vi "DJ Interface.vi"(10 "Owning VI":refnum<vi>, 11 "Shutdown Event":refnum<user-event>) -> ()   [LabVIEW 2020, in "User Interface.lvlib"]
doc: "Main control interface to Dataflow DJ. Also handles all keyboard shortcuts.\n\n<b>Execution System:</b> User Interface"
uses:
  User Interface.lvlib
  Custom Graphics/LED.Red.16px.ctl
  Custom Graphics/Slide.PlaybackPosition.ctl
  Custom Graphics/WaveformGraph.WaveformDisplay.ctl
  Custom Graphics/Knob.276px_Hole.ctl
  Custom Graphics/Button.Large.ctl
  Custom Graphics/PictRing.DeckLabel.ctl
  Custom Graphics/Button.Small.ctl
  <vilib>/Utility/miscctls.llb/LVCursorListTypeDef.ctl
  Packed Libraries/Audio Processing.lvlibp/Value Properties.ctl
  Packed Libraries/Messaging.lvlibp/Message Cluster.ctl
  Controls/Keyboard Shortcut.ctl
  Knob Fill.vi
  <vilib>/Utility/Data Type/Get Type Information.vi
  Packed Libraries/Messaging.lvlibp
  user32.dll
  Packed Libraries/Audio Processing.lvlibp
panel:
  in  "Deck1.Pitch":cluster{dbl, dbl}(slide) scale=30.0..-30.0
  in  "Channel2.EQMidKill":T1
  in  "Channel2.EQLowKill":T1
  in  "Channel2.EQHighKill":T1
  in  "Channel1.EQHighKill":T1
  in  "Channel1.EQMidKill":T1
  in  "Channel1.EQLowKill":T1
  in  "EffectUnit2.Effect3.Value2":dbl(knob) caption="DELAY" scale=0.0..1.0
  in  "EffectUnit2.Effect3.Value1":dbl(knob) caption="AMOUNT" scale=0.0..1.0
  in  "EffectUnit2.Effect2.Value2":dbl(knob)=16.0 caption="BIT DEPTH" step=1.0 scale=0.0..16.0
  in  "EffectUnit2.Effect2.Value1":dbl(knob)=1.0 caption="DECIMATION" step=1.0 scale=1.0..20.0
  in  "EffectUnit2.Effect1.Value2":dbl(knob) caption="SPEED" scale=0.0..0.1
  in  "EffectUnit2.Effect1.Value1":dbl(knob) caption="AMOUNT" scale=0.0..1.0
  in  "EffectUnit1.Effect3.Value2":dbl(knob) caption="DELAY" scale=0.0..1.0
  in  "EffectUnit1.Effect3.Value1":dbl(knob) caption="AMOUNT" scale=0.0..1.0
  in  "EffectUnit1.Effect2.Value2":dbl(knob)=16.0 caption="BIT DEPTH" step=1.0 scale=0.0..16.0
  in  "EffectUnit1.Effect2.Value1":dbl(knob)=1.0 caption="DECIMATION" step=1.0 scale=1.0..20.0
  in  "EffectUnit1.Effect1.Value2":dbl(knob) caption="SPEED" scale=0.0..0.1
  in  "EffectUnit1.Effect1.Value1":dbl(knob) caption="AMOUNT" scale=0.0..1.0
  in  "Channel2.EQLow":dbl(knob)=1.0 caption="LOW" scale=0.0..2.0
  in  "Channel2.EQMid":dbl(knob)=1.0 caption="MID" scale=0.0..2.0
  in  "Channel2.EQHigh":dbl(knob)=1.0 caption="HIGH" scale=0.0..2.0
  in  "Channel2.EQFilter":dbl(knob) caption="FILTER" scale=-1.025..1.025
  in  "Channel1.EQLow":dbl(knob)=1.0 caption="LOW" scale=0.0..2.0
  in  "Channel1.EQMid":dbl(knob)=1.0 caption="MID" scale=0.0..2.0
  in  "Channel1.EQHigh":dbl(knob)=1.0 caption="HIGH" scale=0.0..2.0
  in  "Channel1.EQFilter":dbl(knob) caption="FILTER" scale=-1.025..1.025
  in  "Channel2.Gain":dbl(knob)=1.0 caption="GAIN" scale=0.0..2.0
  in  "Mixer.Headphones":dbl(knob)=1.0 caption="PHONES" scale=0.0..1.0
  in  "Mixer.Master":dbl(knob)=1.0 caption="MASTER" scale=0.0..1.0
  in  "Channel1.Gain":dbl(knob)=1.0 caption="GAIN" scale=0.0..2.0
  out "Default Value Map":variant=variant("Channel1.EQFilter"=variant(dbl 0.0), "Channel1.EQHigh"=variant(dbl 1.0), "Channel1.EQLow"=variant(dbl 1.0), "Channel1.EQMid"=variant(dbl 1.0), "Channel1.Gain"=variant(dbl 1.0), "Channel1.Level"=variant(dbl 1.0), "Channel2.EQFilter"=variant(dbl 0.0), "Channel2.EQHigh"=variant(dbl 1.0), "Channel2.EQLow"=variant(dbl 1.0), "Channel2.EQMid"=variant(dbl 1.0), "Channel2.Gain"=variant(dbl 1.0), "Channel2.Level"=variant(dbl 1.0), "Deck1.Pitch"=variant(dbl 0.0), "Deck2.Pitch"=variant(dbl 0.0), "EffectUnit1.Effect1.Value1"=variant(dbl 0.0), "EffectUnit1.Effect1.Value2"=variant(dbl 0.0), "EffectUnit1.Effect2.Value1"=variant(dbl 1.0), "EffectUnit1.Effect2.Value2"=variant(dbl 16.0), "EffectUnit1.Effect3.Value1"=variant(dbl 0.0), "EffectUnit1.Effect3.Value2"=variant(dbl 0.0), "EffectUnit2.Effect1.Value1"=variant(dbl 0.0), "EffectUnit2.Effect1.Value2"=variant(dbl 0.0), "EffectUnit2.Effect2.Value1"=variant(dbl 1.0), "EffectUnit2.Effect2.Value2"=variant(dbl 16.0), "EffectUnit2.Effect3.Value1"=variant(dbl 0.0), "EffectUnit2.Effect3.Value2"=variant(dbl 0.0), "Mixer.Crossfader"=variant(dbl 0.0), "Mixer.Headphones"=variant(dbl 1.0), "Mixer.Master"=variant(dbl 1.0))
  in  "EffectUnit2.Effect3.Enable":T1
  in  "EffectUnit2.Effect2.Enable":T1
  in  "EffectUnit2.Effect1.Enable":T1
  in  "EffectUnit1.Effect3.Enable":T1
  in  "EffectUnit1.Effect2.Enable":T1
  in  "EffectUnit1.Effect1.Enable":T1
  in  "EffectUnit2.Effect3":u16(ring)=1 items=["CRUSHER", "ECHO", "FLANGER"]
  in  "EffectUnit2.Effect2":u16(ring) items=["CRUSHER", "ECHO", "FLANGER"]
  in  "EffectUnit2.Effect1":u16(ring)=2 items=["CRUSHER", "ECHO", "FLANGER"]
  in  "EffectUnit1.Effect3":u16(ring)=1 items=["CRUSHER", "ECHO", "FLANGER"]
  in  "EffectUnit1.Effect2":u16(ring) items=["CRUSHER", "ECHO", "FLANGER"]
  in  "EffectUnit1.Effect1":u16(ring)=2 items=["CRUSHER", "ECHO", "FLANGER"]
  in  "Deck2.DragDropPath":path
  in  "Deck1.DragDropPath":path
  in  "Deck2.PitchBendUp":T2
  in  "Deck2.PitchBendDown":T2
  in  "Channel2.HeadphoneOutput":T2
  in  "Channel1.HeadphoneOutput":T2
  in  "Deck1.PitchBendUp":T2
  in  "Deck1.PitchBendDown":T2
  in  "Deck2.Reverse":T3
  in  "Deck2.Backspin":T3
  in  "Deck2.Brake":T3
  in  "Deck2.Cue3":T3
  in  "Deck2.Cue2":T3
  in  "Deck2.Cue1":T3
  in  "Deck2.Play":T3
  in  "Deck1.Cue3":T3
  in  "Deck1.Cue2":T3
  in  "Deck1.Reverse":T3
  in  "Deck1.Backspin":T3
  in  "Deck1.Cue1":T3
  out "Deck2.Time":string
  in  "Deck2.PlaybackPosition":T4 scale=0.0..12805632.0
  out "Deck2.Waveform":T5
  out "Deck2.BPM":string
  out "Deck1.BPM":string
  in  "Deck1.Brake":T3
  out "Mixer.Right.LevelIndicator":u8(slide) scale=0.0..20.0
  out "Mixer.Left.LevelIndicator":u8(slide) scale=0.0..20.0
  in  "Deck1.Play":T3
  in  "Deck1.Jogwheel":T6 scale=0.0..79380.0
  in  "Deck2.Pitch":cluster{dbl, dbl}(slide) scale=30.0..-30.0
  out "Deck2.Title":string
  out "Deck1.Time":string
  out "Deck1.Title":string
  in  "Deck2.Jogwheel":T6 scale=0.0..79380.0
  in  "Channel2.Level":dbl(slide)=1.0 scale=0.0..1.0
  in  "Mixer.Crossfader":cluster{dbl, dbl}(slide) scale=-1.0..1.0
  in  "Channel1.Level":dbl(slide)=1.0 scale=0.0..1.0
  in  "Deck1.PlaybackPosition":T4 scale=0.0..12178944.0
  out "Deck1.Waveform":T5
  out "Deck1.JogwheelLabel":T7
  out "Deck2.JogwheelLabel":T7
  # "DECK 1\nCUE"
  # "DECK 2\nCUE"
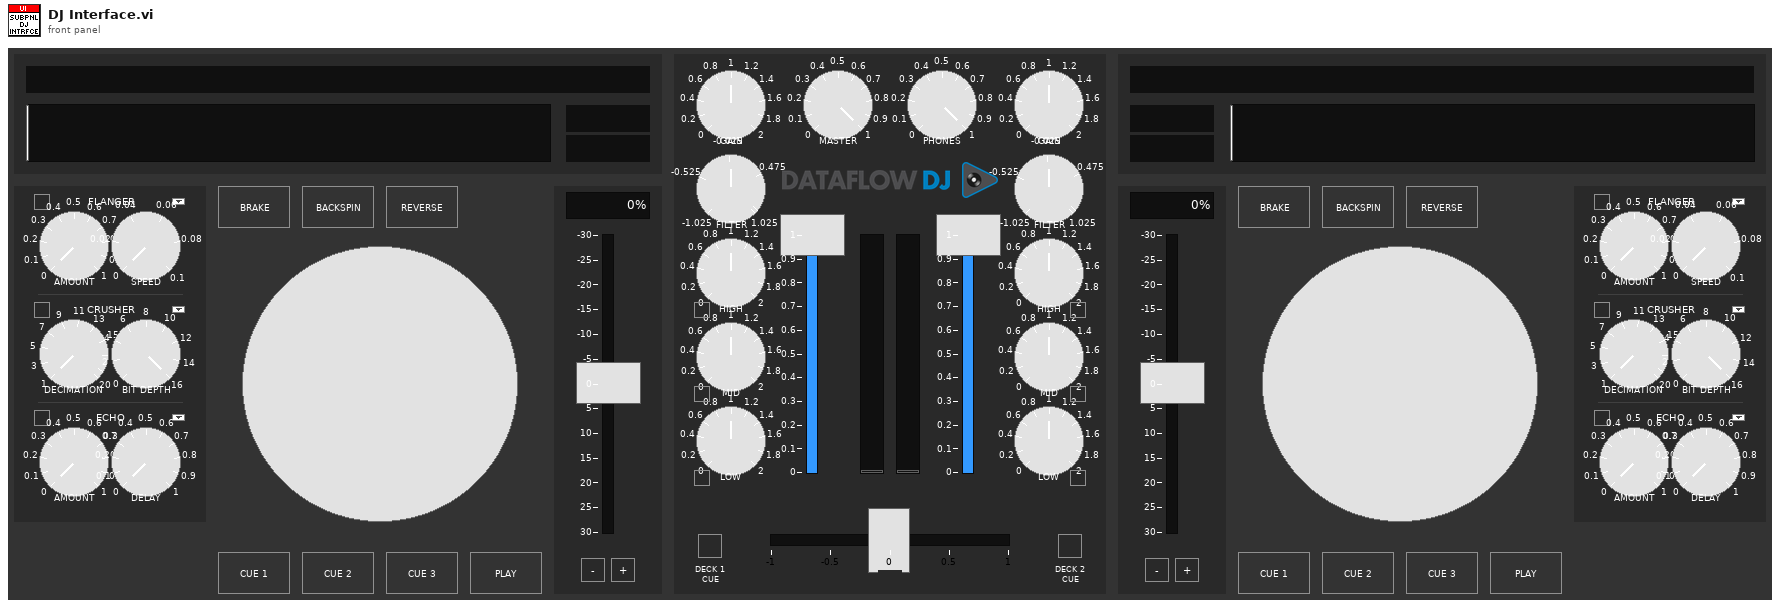
[diagram p1: front panel]
types:
  T1 = typedef "User Interface.lvlib/LED.Red.16px.ctl" = bool
  T2 = typedef "User Interface.lvlib/Button.Small.ctl" = bool
  T3 = typedef "User Interface.lvlib/Button.Large.ctl" = bool
  T4 = typedef "User Interface.lvlib/Slide.PlaybackPosition.ctl" = i32
  T5 = typedef "User Interface.lvlib/WaveformGraph.WaveformDisplay.ctl" = dbl[][]
  T6 = typedef "User Interface.lvlib/Knob.276px_Hole.ctl" = i32
  T7 = typedef "User Interface.lvlib/PictRing.DeckLabel.ctl" = u16
  T8 = typedef "LVCursorListTypeDef.ctl" = cluster{"Name":string, "Color":u32, "Style":u8, "Point Style":u8, "Name Visible":bool, "Allow Drag":bool, "Cursor Mode":u32, "Plot":i32, "Index":i32, "Position":cluster{"X":dbl, "Y":dbl}, "X Scale":u32, "Y Scale":u32, "Watch Plots":i32[], "Watch All Plots":bool, "Plot Area":i32, "Label Offset":cluster{"X":dbl, "Y":dbl}}[]
  T9 = typedef "Keyboard Shortcut.ctl" = cluster{"Keystroke":string, "Message Queue":string, "Event":string, "Target":string, "Data":variant}
  T10 = typedef "Audio Processing.lvlibp/Value Properties.ctl" = cluster{"Lower":dbl, "Upper":dbl, "Default":dbl, "Increment":dbl}
  T11 = typedef "Messaging.lvlib/Message Cluster.ctl" = cluster{"Event":string, "Source":string, "Target":string, "Data":variant}
  T12 = typedef "Messaging.lvlibp/Message Cluster.ctl" = cluster{"Event":string, "Source":string, "Target":string, "Data":variant}
  T13 = cluster{"type":i32, "KEYBDINPUT":cluster{"dx":i32, "dy":i32, "mouseData":i32, "dwFlags":i32, "time":i32, "dwExtraInfo":u32}}
  T14 = typedef "eventvkey.ctl" = enum16{"ASCII", "Enter", "Return", "Shift", "Ctrl", "Alt", "Cmd", "Opt", "Caps", "NumLock", "Clear", "Break", "Up", "Down", "Left", "Right", "Insert", "Delete", "Home", "End", "PageUp", "PageDown", "Escape", "Help", "Pause", "ScrollLock", "F1", "F2", "F3", "F4", "F5", "F6", "F7", "F8", "F9", "F10", "F11", "F12", "F13", "F14", "F15", "F16", "F17", "F18", "F19", "F20", "F21", "F22", "F23", "F24", "Play", "VolumeUp", "VolumeDown", "Mute", "Two Byte Char"}
  T15 = cluster{"Shift":bool, "Ctrl":bool, "Alt":bool, "Cmd":bool, "Opt":bool}
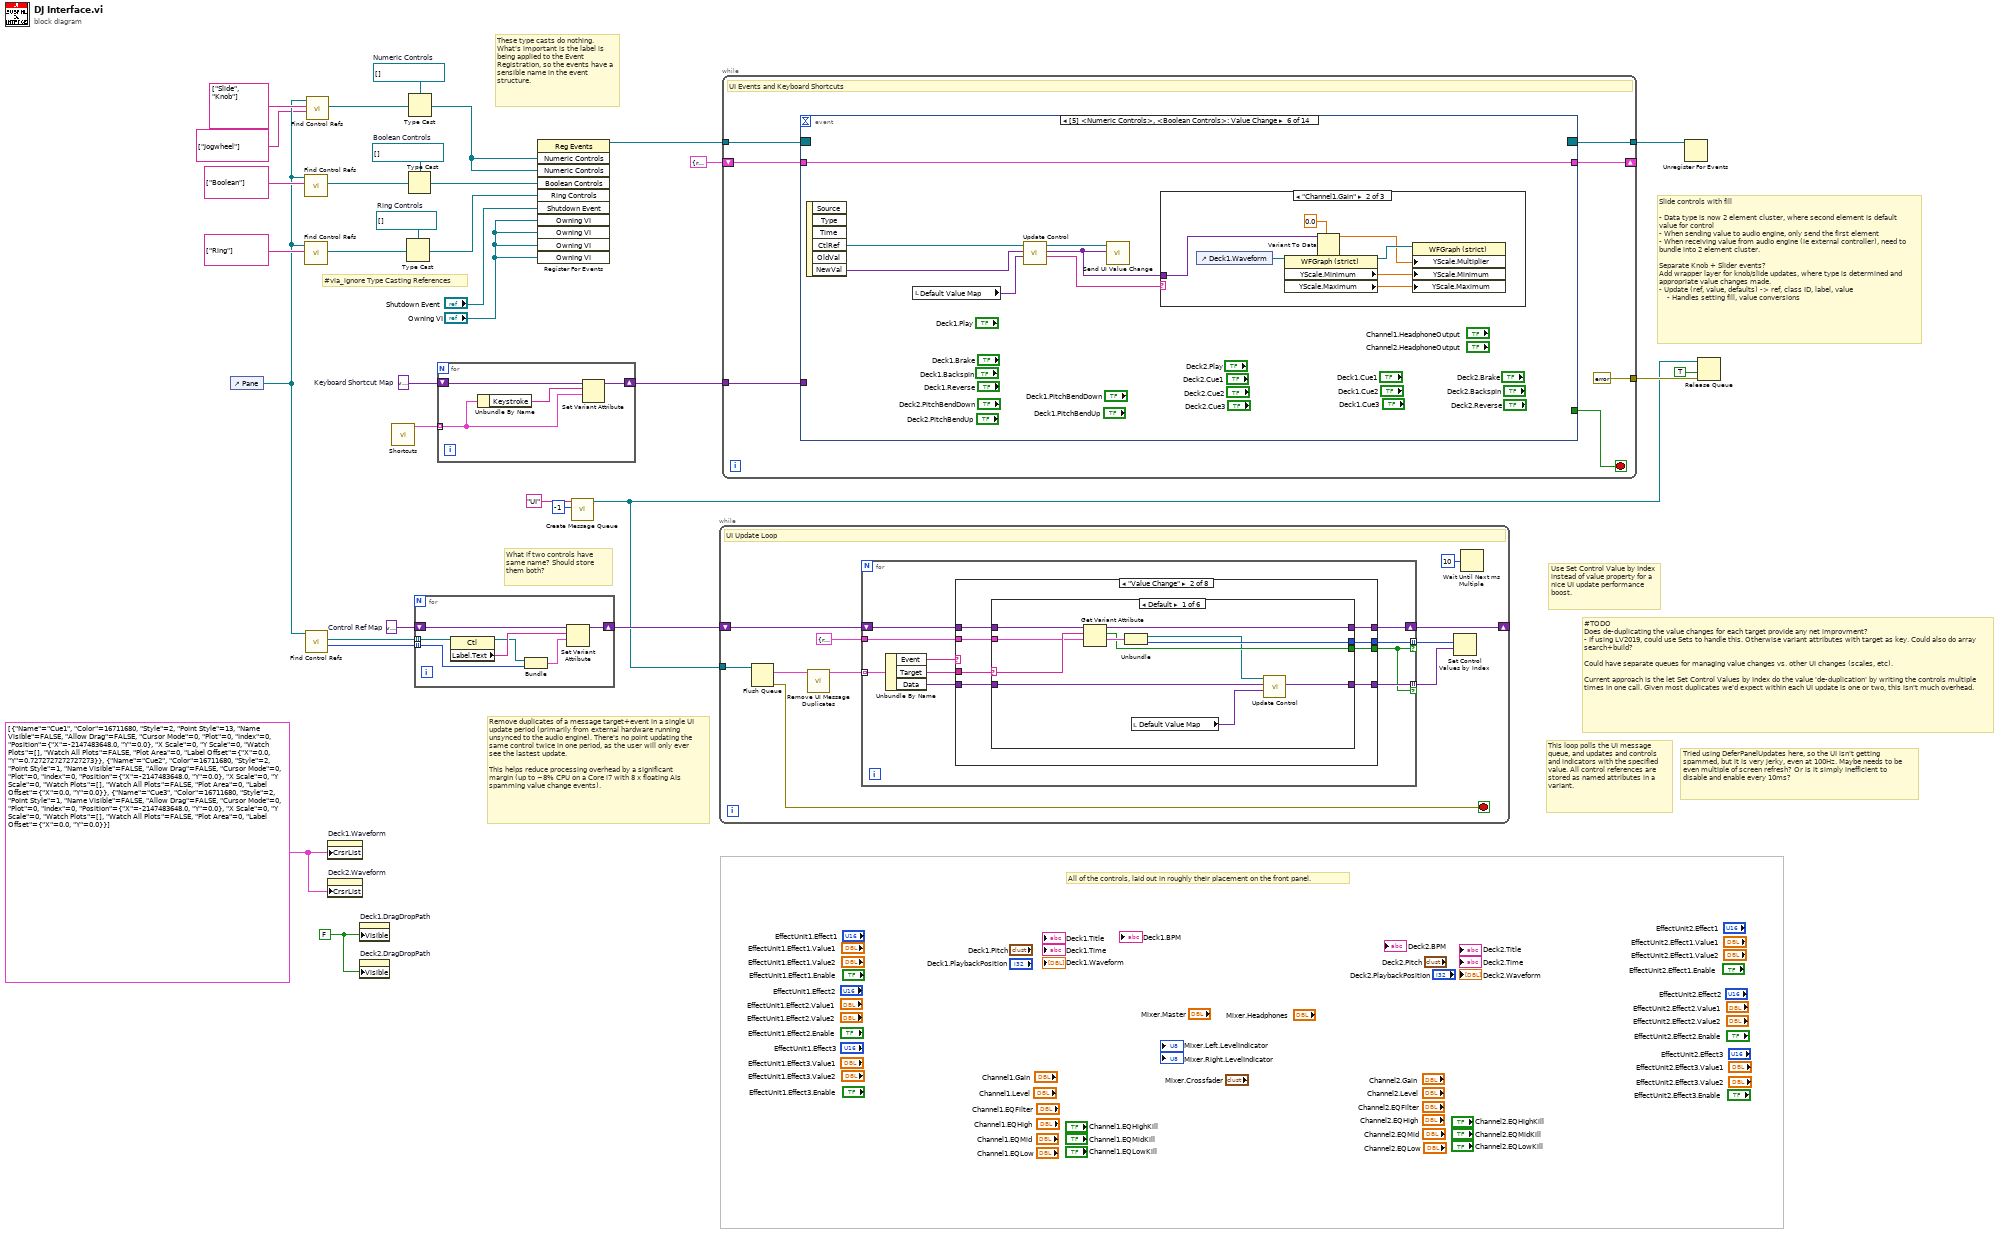
[diagram p0: block diagram]
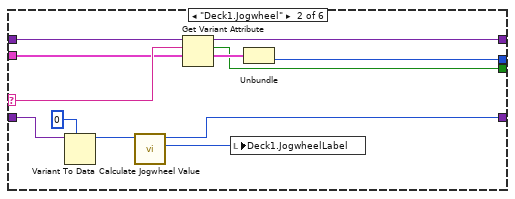
[diagram p3: hidden frame]
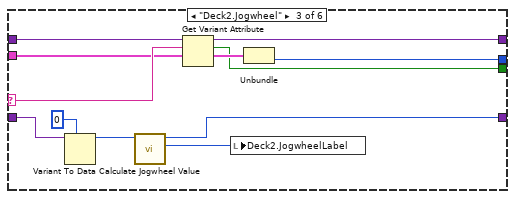
[diagram p4: hidden frame]
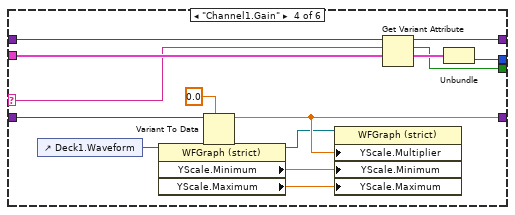
[diagram p5: hidden frame]
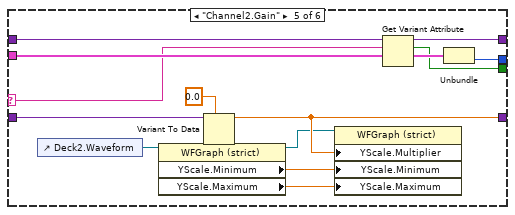
[diagram p6: hidden frame]
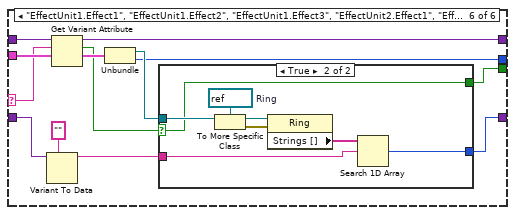
[diagram p7: hidden frame]
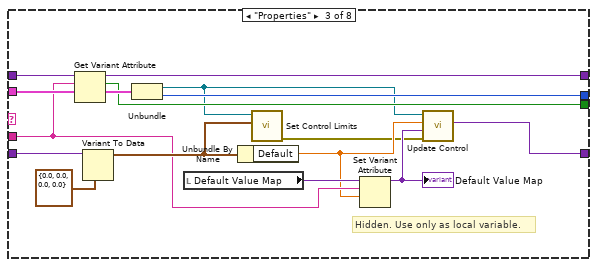
[diagram p9: hidden frame]
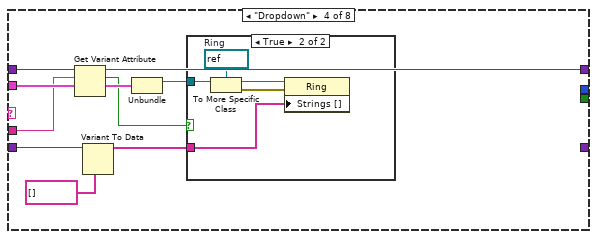
[diagram p10: hidden frame]
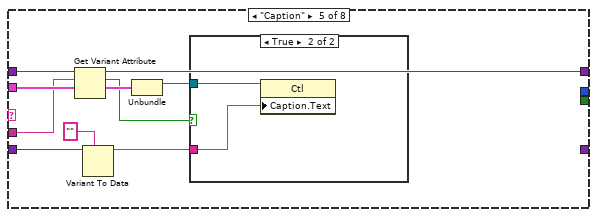
[diagram p12: hidden frame]
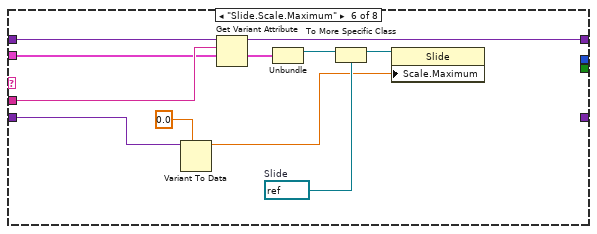
[diagram p14: hidden frame]
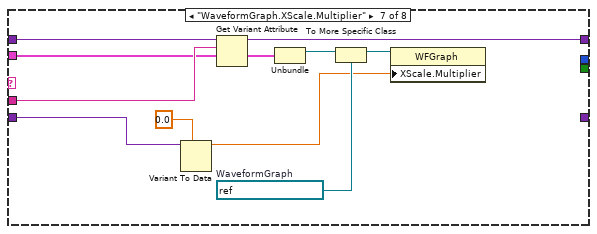
[diagram p15: hidden frame]
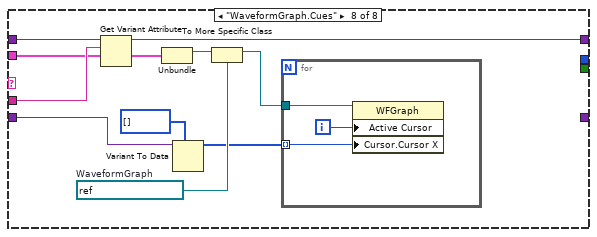
[diagram p16: hidden frame]
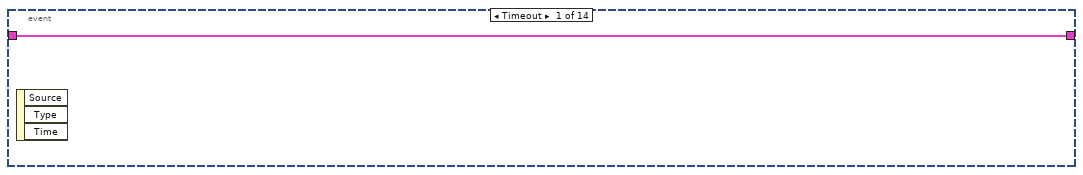
[diagram p17: hidden frame]
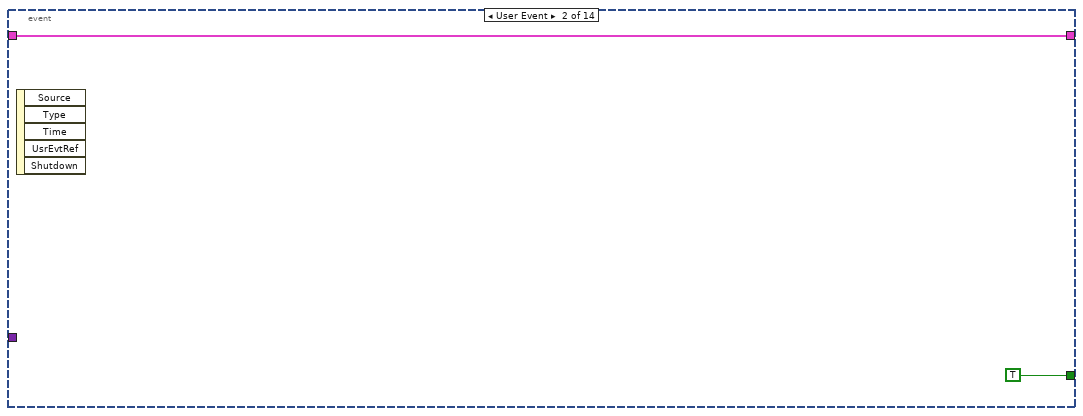
[diagram p18: hidden frame]
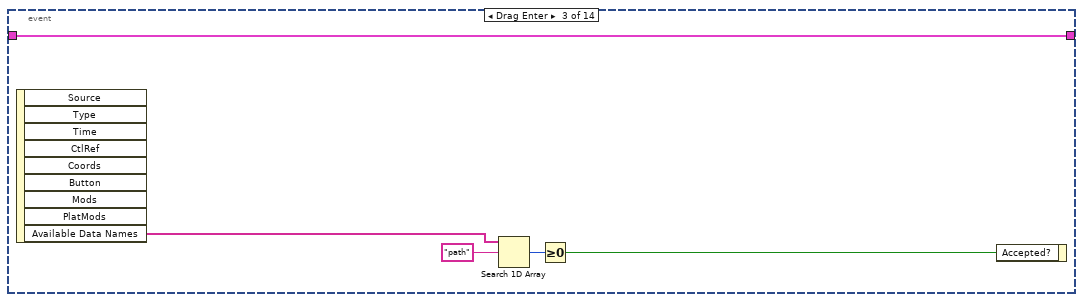
[diagram p19: hidden frame]
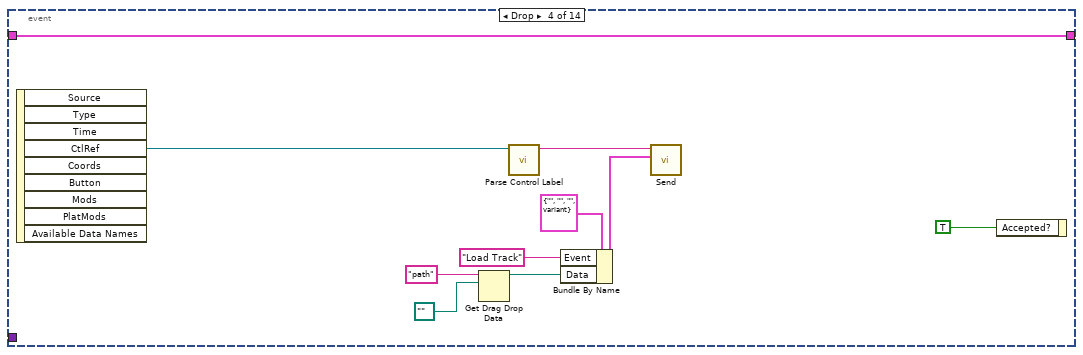
[diagram p20: hidden frame]
diagram:
  w6 = refnum<vi>[] []  # Ring Controls
  w10 = FALSE ("Visible")
  w12 = T8 [{"Name"="Cue1", "Color"=16711680, "Style"=2, "Point Style"=13, "Name Visible"=FALSE, "Allow Drag"=FALSE, "Cursor Mode"=0, "Plot"=0, "Index"=0, "Position"={"X"=-2147483648.0, "Y"=0.0}, "X Scale"=0, "Y Scale"=0, "Watch Plots"=[], "Watch All Plots"=FALSE, "Plot Area"=0, "Label Offset"={"X"=0.0, "Y"=0.7272727272727273}}, {"Name"="Cue2", "Color"=16711680, "Style"=2, "Point Style"=1, "Name Visible"=FALSE, "Allow Drag"=FALSE, "Cursor Mode"=0, "Plot"=0, "Index"=0, "Position"={"X"=-2147483648.0, "Y"=0.0}, "X Scale"=0, "Y Scale"=0, "Watch Plots"=[], "Watch All Plots"=FALSE, "Plot Area"=0, "Label Offset"={"X"=0.0, "Y"=0.0}}, {"Name"="Cue3", "Color"=16711680, "Style"=2, "Point Style"=1, "Name Visible"=FALSE, "Allow Drag"=FALSE, "Cursor Mode"=0, "Plot"=0, "Index"=0, "Position"={"X"=-2147483648.0, "Y"=0.0}, "X Scale"=0, "Y Scale"=0, "Watch Plots"=[], "Watch All Plots"=FALSE, "Plot Area"=0, "Label Offset"={"X"=0.0, "Y"=0.0}}] ("Cursor List")
  w25 = variant  # Keyboard Shortcut Map
  w28 = variant  # Control Ref Map
  w32 = refnum<vi>[] []  # Boolean Controls
  w31 = refnum<vi>[] []  # Numeric Controls
  # "Remove duplicates of a message target+event in a single UI update period (primarily from external hardware running unsynced to the audio engine). There's no point updating the same control twice in one period, as the user will only ever see the lastest update.\n\nThis helps reduce processing overhead by a significant margin (up to ~8% CPU on a Core i7 with 8 x floating AIs spamming value change events)."
  # "Slide controls with fill\n\n- Data type is now 2 element cluster, where second element is default value for control\n- When sending value to audio engine, only send the first element\n- When receiving value from audio engine (ie external controller), need to bundle into 2 element cluster.\n\nSeparate Knob + Slider events?\nAdd wrapper layer for knob/slide updates, where type is determined and appropriate value changes made.\n- Update (ref, value, defaults) -> ref, class ID, label, value\n    - Handles setting fill, value conversions"
  # "#via_ignore Type Casting References"
  # "Use Set Control Value by Index instead of value property for a nice UI update performance boost."
  # "#TODO\nDoes de-duplicating the value changes for each target provide any net improvment?\n- If using LV2019, could use Sets to handle this. Otherwise variant attributes with target as key. Could also do array search+build?\n\nCould have separate queues for managing value changes vs. other UI changes (scales, etc).\n\nCurrent approach is the let Set Control Values by Index do the value 'de-duplication' by writing the controls multiple times in one call. Given most duplicates we'd expect within each UI update is one or two, this isn't much overhead."
  # "What if two controls have same name? Should store them both?"
  # "All of the controls, laid out in roughly their placement on the front panel."
  # "This loop polls the UI message queue, and updates and controls and indicators with the specified value. All control references are stored as named attributes in a variant."
  # "Tried using DeferPanelUpdates here, so the UI isn't getting spammed, but it is very jerky, even at 100Hz. Maybe needs to be even multiple of screen refresh? Or is it simply inefficient to disable and enable every 10ms?"
  # "These type casts do nothing. What's important is the label is being applied to the Event Registration, so the events have a sensible name in the event structure."
  n1 = control-ref of="Pane"() -> (w2:refnum<vi>)
  n2 = call "Find Control Refs.vi"("Control Types"=string[] ["Boolean"], "Pane Reference In"=w2) -> ("Control Refs"=w16:refnum<vi>[])  [unwired: 7 in, 2 out]
  n3 = call "Find Control Refs.vi"("Control Types"=string[] ["Ring"], "Pane Reference In"=w2) -> ("Control Refs"=w5:refnum<vi>[])  [unwired: 7 in, 2 out]
  n4 = call "Find Control Refs.vi"("Pane Reference In"=w2) -> ("Control Indicies"=w8:i32[], "Control Refs"=w15:refnum<vi>[])  [unwired: 8 in, 1 out]
  n5 = call "Find Control Refs.vi"("Label.Text Filter"=string[] ["Jogwheel"], "Control Types"=string[] ["Slide", "Knob"], "Pane Reference In"=w2) -> ("Control Refs"=w9:refnum<vi>[])  [unwired: 6 in, 2 out]
  n6 = property on="Deck1.Waveform" class="WFGraph (strict)"("CrsrList"=w12) -> ()  [unwired: 2 in, 2 out]
  n7 = property on="Deck2.Waveform" class="WFGraph (strict)"("CrsrList"=w12) -> ()  [unwired: 2 in, 2 out]
  n8 = property on="Deck1.DragDropPath" class="Path"("Visible"=w10) -> ()  [unwired: 2 in, 2 out]
  n9 = property on="Deck2.DragDropPath" class="Path"("Visible"=w10) -> ()  [unwired: 2 in, 2 out]
  n10 = call "Shortcuts.vi"() -> ("Keyboard Shortcuts"=w23:T9[])  [unwired: 11 in]
  n11 = Type Cast(type=w6, x=w5) -> (*(type *) &x=w4:refnum<vi>[])
  n12 = Type Cast(type=w32, x=w16) -> (*(type *) &x=w29:refnum<vi>[])
  n13 = Type Cast(type=w31, x=w9) -> (*(type *) &x=w14:refnum<vi>[])
  n14 = for {
    shift-right: [w39] -> w27
    shift-left: w28 -> [w40]
    tunnel: w15 -> [w38] mode=indexing
    tunnel: w8 -> [w35] mode=indexing
    n15 = property class="Ctl"(reference=w38) -> (reference out=w36:refnum<vi>, "Label.Text"=w37:string)  [unwired: 1 in, 1 out]
    n16 = Bundle(w36, w35) -> (w34:cluster{refnum<vi>, i32})  [unwired: 1 in]
    n17 = Set Variant Attribute(Variant=w40, name=w37, value=w34) -> (Variant out=w39:variant)  [unwired: 1 in, 2 out]
  }
  n18 = for {
    shift-right: [w43] -> w24
    shift-left: w25 -> [w44]
    tunnel: w23 -> [w41] mode=indexing
    n19 = Unbundle By Name(w41) -> ("Keystroke"=w42:string)
    n20 = Set Variant Attribute(Variant=w44, name=w42, value=w41) -> (Variant out=w43:variant)  [unwired: 1 in, 2 out]
  }
  n21 = register-events(w14, w14, w29, w4, "Shutdown Event", "Owning VI", "Owning VI", "Owning VI", "Owning VI") -> (reference out=w33:refnum<event-registration>)  [unwired: 2 in, 1 out]
  n22 = call "Create Message Queue.vi"("Max Size (1000)"=-1, "Queue Name"="UI") -> ("queue out"=w19:refnum<queue>)  [unwired: 8 in, 1 out]
  n23 = while {
    tunnel: w19 -> [w52]
    shift-right: [w53] -> _
    shift-left: w27 -> [w54]
    stop <- w50 stop-if-true
    # "UI Update Loop"
    n24 = Flush Queue(queue=w52) -> (remaining elements=w46:T11[], error out=w50:errorcluster)  [unwired: 1 in, 1 out]
    n25 = call "Remove UI Message Duplicates.vi"("Messages In"=w46) -> ("Messages Out"=w45:T12[])  [unwired: 10 in]
    n26 = for {
      shift-right: [w63] -> w53
      shift-left: w54 -> [w64]
      tunnel: w45 -> [w59] mode=indexing
      tunnel: cluster{refnum<vi>, i32} {refnum, 0} ("output cluster") -> [w58]
      tunnel: [w57] -> w48 mode=indexing if=w55
      tunnel: [w56] -> w47 mode=indexing if=w55
      n27 = Unbundle By Name(w59) -> ("Event"=w62:string, "Target"=w60:string, "Data"=w61:variant)
      n28 = case shown="\"Value Change\"" w62 {
        tunnel: w64 -> [w66 w74 w172 w183 w197 w213 w224 w235]
        tunnel: w60 -> [_ w71 w165 w180 w194 w211 w222 w233]
        tunnel: [w66 w73 w171 w182 w196 w212 w223 w234] -> w63
        tunnel: w61 -> [w65 w72 w174 w185 w199 w207 w218 w229]
        tunnel: w58 -> [_ w70 w169 w181 w195 w205 w216 w227]
        tunnel: [_ w69 w170 _ _ _ _ _] -> w57
        tunnel: [_ w67 w168 _ _ _ _ _] -> w55
        tunnel: [w65 w68 w161 _ _ _ _ _] -> w56
        frame Default {
        }
        frame "Value Change" {
          n29 = case shown="Default" w71 {
            selector: w71 -> [w83 w95 w107 w114 w128 w147]
            tunnel: w74 -> [w85 w97 w109 w123 w137 w149]
            tunnel: [w84 w96 w108 w122 w136 w146] -> w73
            tunnel: w72 -> [w77 w94 w106 w116 w130 w143]
            tunnel: w70 -> [w82 w90 w102 w120 w134 w148]
            tunnel: [w80 w87 w99 w118 w132 w139] -> w69
            tunnel: [w76 w89 w101 w111 w125 w140] -> w68
            tunnel: [w79 w86 w98 w117 w131 w138] -> w67
            frame Default {
              n30 = Get Variant Attribute(Variant=w85, name=w83, default value (empty Variant)=w82) -> (duplicate Variant=w84:variant, found=w79:bool, value=w81:cluster{refnum<vi>, i32})  [unwired: 1 in, 1 out]
              n31 = Unbundle(w81) -> (w78:refnum<vi>, w80:i32)
              n32 = local read "Default Value Map"() -> (w75:variant)
              n33 = call "Update Control.vi"("Default Value Map"=w75, "Value In"=w77, "Control Ref"=w78) -> ("Value Out"=w76:variant)  [unwired: 5 in, 3 out]
            }
            frame "Deck1.Jogwheel" {
              n34 = Variant To Data(type=0 ("y"), Variant=w94) -> (data=w92:i32)  [unwired: 1 in, 1 out]
              n35 = call "Calculate Jogwheel Value.vi"("Playback Position"=w92) -> ("Jogwheel Label Image"=w91:i32, "Jogwheel Position"=w89:i32)  [unwired: 9 in]
              n36 = Get Variant Attribute(Variant=w97, name=w95, default value (empty Variant)=w90) -> (duplicate Variant=w96:variant, found=w86:bool, value=w88:cluster{refnum<vi>, i32})  [unwired: 1 in, 1 out]
              n37 = local write "Deck1.JogwheelLabel"(w91) -> ()
              n38 = Unbundle(w88) -> (w87:i32)  [unwired: 1 out]
            }
            frame "Deck2.Jogwheel" {
              n39 = Variant To Data(type=0 ("y"), Variant=w106) -> (data=w104:i32)  [unwired: 1 in, 1 out]
              n40 = call "Calculate Jogwheel Value.vi"("Playback Position"=w104) -> ("Jogwheel Label Image"=w103:i32, "Jogwheel Position"=w101:i32)  [unwired: 9 in]
              n41 = Get Variant Attribute(Variant=w109, name=w107, default value (empty Variant)=w102) -> (duplicate Variant=w108:variant, found=w98:bool, value=w100:cluster{refnum<vi>, i32})  [unwired: 1 in, 1 out]
              n42 = local write "Deck2.JogwheelLabel"(w103) -> ()
              n43 = Unbundle(w100) -> (w99:i32)  [unwired: 1 out]
            }
            frame "Channel1.Gain" {
              n44 = control-ref of="Deck1.Waveform"() -> (w115:refnum<vi>)
              n45 = property class="WFGraph (strict)"(reference=w115) -> (reference out=w110:refnum<vi>, "YScale.Minimum"=w113:dbl, "YScale.Maximum"=w112:dbl)  [unwired: 1 in, 1 out]
              n46 = Variant To Data(type=0.0 ("y"), Variant=w116) -> (data=w111:dbl)  [unwired: 1 in, 1 out]
              n47 = property class="WFGraph (strict)"(reference=w110, "YScale.Multiplier"=w111, "YScale.Minimum"=w113, "YScale.Maximum"=w112) -> ()  [unwired: 1 in, 2 out]
              n48 = Get Variant Attribute(Variant=w123, name=w114, default value (empty Variant)=w120) -> (duplicate Variant=w122:variant, found=w117:bool, value=w119:cluster{refnum<vi>, i32})  [unwired: 1 in, 1 out]
              n49 = Unbundle(w119) -> (w118:i32)  [unwired: 1 out]
            }
            frame "Channel2.Gain" {
              n50 = control-ref of="Deck2.Waveform"() -> (w129:refnum<vi>)
              n51 = property class="WFGraph (strict)"(reference=w129) -> (reference out=w124:refnum<vi>, "YScale.Minimum"=w127:dbl, "YScale.Maximum"=w126:dbl)  [unwired: 1 in, 1 out]
              n52 = Variant To Data(type=0.0 ("y"), Variant=w130) -> (data=w125:dbl)  [unwired: 1 in, 1 out]
              n53 = property class="WFGraph (strict)"(reference=w124, "YScale.Multiplier"=w125, "YScale.Minimum"=w127, "YScale.Maximum"=w126) -> ()  [unwired: 1 in, 2 out]
              n54 = Get Variant Attribute(Variant=w137, name=w128, default value (empty Variant)=w134) -> (duplicate Variant=w136:variant, found=w131:bool, value=w133:cluster{refnum<vi>, i32})  [unwired: 1 in, 1 out]
              n55 = Unbundle(w133) -> (w132:i32)  [unwired: 1 out]
            }
            frame "EffectUnit1.Effect1", "EffectUnit1.Effect2", "EffectUnit1.Effect3", "EffectUnit2.Effect1", "EffectUnit2.Effect2", "EffectUnit2.Effect3" {
              n56 = Variant To Data(type="", Variant=w143) -> (data=w141:string)  [unwired: 1 in, 1 out]
              n57 = Get Variant Attribute(Variant=w149, name=w147, default value (empty Variant)=w148) -> (duplicate Variant=w146:variant, found=w145:bool, value=w150:cluster{refnum<vi>, i32})  [unwired: 1 in, 1 out]
              n58 = Unbundle(w150) -> (w144:refnum<vi>, w139:i32)
              n59 = case shown="True" w145 {
                selector: w145 -> [w151 w152]
                tunnel: w144 -> [_ w159]
                tunnel: w141 -> [_ w155]
                tunnel: [_ w153] -> w140
                tunnel: [w151 w152] -> w138
                frame False {
                }
                frame True {
                  w158 = refnum<vi> refnum  # Ring
                  n60 = To More Specific Class(target class=w158, reference=w159) -> (specific class reference=w157:refnum<vi>, error out=w154:errorcluster)  [unwired: 1 in]
                  n61 = property class="Ring"(reference=w157, error in=w154) -> ("Strings []"=w156:string[])  [unwired: 2 out]
                  n62 = Search 1D Array(1D array=w156, element=w155) -> (index of element=w153:i32)  [unwired: 1 in]
                }
              }
            }
          }
        }
        frame "Properties" {
          # "Hidden. Use only as local variable."
          n63 = Get Variant Attribute(Variant=w172, name=w165, default value (empty Variant)=w169) -> (duplicate Variant=w171:variant, found=w168:bool, value=w173:cluster{refnum<vi>, i32})  [unwired: 1 in, 1 out]
          n64 = Variant To Data(type=T10 {"Lower"=0.0, "Upper"=0.0, "Default"=0.0, "Increment"=0.0} ("Value Properties"), Variant=w174) -> (data=w167:T10)  [unwired: 1 in, 1 out]
          n65 = Unbundle(w173) -> (w164:refnum<vi>, w170:i32)
          n66 = local read "Default Value Map"() -> (w166:variant)
          n67 = Unbundle By Name(w167) -> ("Default"=w163:dbl)
          n68 = call "Set Control Limits.vi"("Value Properties"=w167, "Control Ref"=w164) -> ("error out"=w160:errorcluster)  [unwired: 9 in]
          n69 = Set Variant Attribute(Variant=w166, name=w165, value=w163) -> (Variant out=w162:variant)  [unwired: 1 in, 2 out]
          "Default Value Map" <- w162
          n70 = call "Update Control.vi"("error in (no error)"=w160, "Default Value Map"=w162, "Value In"=w163, "Control Ref"=w164) -> ("Value Out"=w161:variant)  [unwired: 4 in, 3 out]
        }
        frame "Dropdown" {
          n71 = Get Variant Attribute(Variant=w183, name=w180, default value (empty Variant)=w181) -> (duplicate Variant=w182:variant, found=w178:bool, value=w184:cluster{refnum<vi>, i32})  [unwired: 1 in, 1 out]
          n72 = Variant To Data(type=string[] [], Variant=w185) -> (data=w176:string[])  [unwired: 1 in, 1 out]
          n73 = Unbundle(w184) -> (w177:refnum<vi>)  [unwired: 1 out]
          n74 = case shown="True" w178 {
            tunnel: w177 -> [_ w190]
            tunnel: w176 -> [_ w187]
            frame False {
            }
            frame True {
              w188 = refnum<vi> refnum  # Ring
              n75 = To More Specific Class(target class=w188, reference=w190) -> (specific class reference=w189:refnum<vi>, error out=w186:errorcluster)  [unwired: 1 in]
              n76 = property class="Ring"(reference=w189, error in=w186, "Strings []"=w187) -> ()  [unwired: 2 out]
            }
          }
        }
        frame "Caption" {
          n77 = Get Variant Attribute(Variant=w197, name=w194, default value (empty Variant)=w195) -> (duplicate Variant=w196:variant, found=w193:bool, value=w198:cluster{refnum<vi>, i32})  [unwired: 1 in, 1 out]
          n78 = Variant To Data(type="", Variant=w199) -> (data=w191:string)  [unwired: 1 in, 1 out]
          n79 = Unbundle(w198) -> (w192:refnum<vi>)  [unwired: 1 out]
          n80 = case shown="True" w193 {
            tunnel: w192 -> [_ w202]
            tunnel: w191 -> [_ w201]
            frame False {
            }
            frame True {
              n81 = property class="Ctl"(reference=w202, "Caption.Text"=w201) -> ()  [unwired: 1 in, 2 out]
            }
          }
        }
        frame "Slide.Scale.Maximum" {
          w210 = refnum<vi> refnum  # Slide
          n82 = Variant To Data(type=0.0, Variant=w207) -> (data=w208:dbl)  [unwired: 1 in, 1 out]
          n83 = Get Variant Attribute(Variant=w213, name=w211, default value (empty Variant)=w205) -> (duplicate Variant=w212:variant, value=w204:cluster{refnum<vi>, i32})  [unwired: 1 in, 2 out]
          n84 = Unbundle(w204) -> (w203:refnum<vi>)  [unwired: 1 out]
          n85 = To More Specific Class(target class=w210, reference=w203) -> (specific class reference=w209:refnum<vi>)  [unwired: 1 in, 1 out]
          n86 = property class="Slide"(reference=w209, "Scale.Maximum"=w208) -> ()  [unwired: 1 in, 2 out]
        }
        frame "WaveformGraph.XScale.Multiplier" {
          w221 = refnum<vi> refnum  # WaveformGraph
          n87 = Variant To Data(type=0.0, Variant=w218) -> (data=w219:dbl)  [unwired: 1 in, 1 out]
          n88 = Get Variant Attribute(Variant=w224, name=w222, default value (empty Variant)=w216) -> (duplicate Variant=w223:variant, value=w215:cluster{refnum<vi>, i32})  [unwired: 1 in, 2 out]
          n89 = Unbundle(w215) -> (w214:refnum<vi>)  [unwired: 1 out]
          n90 = To More Specific Class(target class=w221, reference=w214) -> (specific class reference=w220:refnum<vi>)  [unwired: 1 in, 1 out]
          n91 = property class="WFGraph"(reference=w220, "XScale.Multiplier"=w219) -> ()  [unwired: 1 in, 2 out]
        }
        frame "WaveformGraph.Cues" {
          w232 = refnum<vi> refnum  # WaveformGraph
          n92 = Get Variant Attribute(Variant=w235, name=w233, default value (empty Variant)=w227) -> (duplicate Variant=w234:variant, value=w226:cluster{refnum<vi>, i32})  [unwired: 1 in, 2 out]
          n93 = Unbundle(w226) -> (w225:refnum<vi>)  [unwired: 1 out]
          n94 = Variant To Data(type=i32[] [], Variant=w229) -> (data=w230:i32[])  [unwired: 1 in, 1 out]
          n95 = To More Specific Class(target class=w232, reference=w225) -> (specific class reference=w231:refnum<vi>)  [unwired: 1 in, 1 out]
          n96 = for {
            tunnel: w231 -> [w238]
            tunnel: w230 -> [w237] mode=indexing
            i -> [w236]
            n97 = property class="WFGraph"(reference=w238, "Active Cursor"=w236, "Cursor.Cursor X"=w237) -> ()  [unwired: 1 in, 2 out]
          }
        }
      }
    }
    n98 = Set Control Values by Index(1:w48, 2:w47) -> ()  [unwired: 2 in, 1 out]
    n99 = Wait Until Next ms Multiple(millisecond multiple=u32 10) -> ()  [unwired: 1 out]
  }
  n100 = while {
    tunnel: [errorcluster {"status"=FALSE, "code"=0, "source"=""} ("error in (no error)")] -> w26
    tunnel: w33 -> [w244]
    tunnel: [w243] -> w30
    tunnel: w24 -> [w242]
    shift-right: [w240] -> _
    shift-left: cluster{"CtlRef":refnum<vi>, "Value":variant} {"CtlRef"=refnum, "Value"=variant} -> [w239]
    stop <- w241 stop-if-true
    # "UI Events and Keyboard Shortcuts"
    n101 = event shown="[5] <Numeric Controls>, <Boolean Controls>: Value Change" {
      selector: w244 -> [_ _ _ _ _ _ _ _ _ _ _ _ _ _]
      dyn-events: [_ _ _ _ _ _ _ _ _ _ _ _ _ _] -> w243
      timeout: _ -> [_ _ _ _ _ _ _ _ _ _ _ _ _ _]
      tunnel: w242 -> [_ _ _ _ _ _ _ _ _ _ w360 _ _ _]
      tunnel: [_ TRUE _ _ _ _ _ _ _ _ _ _ _ _] -> w241
      tunnel: [w246 w247 w249 w254 w272 w279 w301 w304 w338 w344 w354 w373 w394 w396] -> w240
      tunnel: w239 -> [w246 w247 w249 w254 w272 w279 w301 w303 w338 w344 w354 w374 w394 w396]
      event Timeout {
        n102 = event-data() -> ()  [unwired: 1 in, 3 out]
      }
      event User Event {
        n103 = event-data() -> ()  [unwired: 1 in, 5 out]
      }
      event Drag Enter {
        n104 = event-data() -> ("Available Data Names"=w251:string[])  [unwired: 1 in, 8 out]
        n105 = Search 1D Array(1D array=w251, element="path") -> (index of element=w252:i32)  [unwired: 1 in]
        n106 = Greater Or Equal To 0?(x=w252) -> (x >= 0?=w250:bool)
        n107 = event-data("Accepted?"=w250) -> ()  [unwired: 1 in, 1 out]
      }
      event Drop {
        n108 = event-data() -> ("CtlRef"=w257:refnum<vi>)  [unwired: 1 in, 8 out]
        n109 = Get Drag Drop Data(8:path "", 9:"path" ("data name")) -> (3:w255:path)  [unwired: 1 in, 1 out]
        n110 = call "Parse Control Label.vi"("CtlRef"=w257) -> ("Queue Name"=w256:string)  [unwired: 9 in, 1 out]
        n111 = Bundle By Name(cluster=T12 {"Event"="", "Source"="", "Target"="", "Data"=variant} ("Message"), "Event"="Load Track" ("Type"), "Data"=w255) -> (w259:T12)
        n112 = call "Send.vi"("Message"=w259, "Queue Name"=w256) -> ()  [unwired: 9 in, 1 out]
        n113 = event-data("Accepted?"=TRUE) -> ()  [unwired: 1 in, 1 out]
      }
      event "Deck1.DragDropPath", "Deck2.DragDropPath": Value Change {
        # "#BUG\nThe path control doesn't reliably receive the drop event (and corresponding value change) when the control is hidden on mouse entry. This only seems to be for one of the path controls (despite number of path controls on FP), and has only been observed on Windows 8 at run-time.\n\nOne workaround is to hide the path controls after a value change, or on mouse release."
        # "Hidden"
        # "Blank the value, otherwise it'll be visible when the mouse leaves the application window again. We already have the value in the event data, so safe to blank out straight away."
        n114 = event-data() -> ("CtlRef"=w266:refnum<vi>, "NewVal"=w267:path)  [unwired: 1 in, 4 out]
        n115 = property class="Path"(reference=w266, "Value"=path "") -> (reference out=w264:refnum<vi>)  [unwired: 1 in, 1 out]
        n116 = call "Parse Control Label.vi"("CtlRef"=w264) -> ("Queue Name"=w271:string)  [unwired: 9 in, 1 out]
        n117 = Bundle By Name(cluster=T12 {"Event"="", "Source"="", "Target"="", "Data"=variant} ("Message"), "Event"="Load Track" ("Type"), "Data"=w267) -> (w269:T12)
        n118 = call "Send.vi"("Message"=w269, "Queue Name"=w271) -> ()  [unwired: 9 in, 1 out]
      }
      event Value Change {
        n119 = event-data() -> ("CtlRef"=w278:refnum<vi>, "NewVal"=w276:variant)  [unwired: 1 in, 4 out]
        n120 = local read "Default Value Map"() -> (w277:variant)
        n121 = call "Update Control.vi"("Default Value Map"=w277, "Value In"=w276, "Control Ref"=w278) -> ("Label Text"=w273:string, "Value Out"=w274:variant, "Control Ref (Dup)"=w275:refnum<vi>)  [unwired: 5 in, 1 out]
        n122 = call "Send UI Value Change.vi"("Data"=w274, "CtlRef"=w275) -> ()  [unwired: 10 in]
        n123 = case shown="\"Channel1.Gain\"" w273 {
          tunnel: w274 -> [_ w281 w288]
          frame Default {
          }
          frame "Channel1.Gain" {
            n124 = control-ref of="Deck1.Waveform"() -> (w285:refnum<vi>)
            n125 = property class="WFGraph (strict)"(reference=w285) -> (reference out=w282:refnum<vi>, "YScale.Minimum"=w284:dbl, "YScale.Maximum"=w283:dbl)  [unwired: 1 in, 1 out]
            n126 = Variant To Data(type=0.0 ("y"), Variant=w281) -> (data=w280:dbl)  [unwired: 1 in, 1 out]
            n127 = property class="WFGraph (strict)"(reference=w282, "YScale.Multiplier"=w280, "YScale.Minimum"=w284, "YScale.Maximum"=w283) -> ()  [unwired: 1 in, 2 out]
          }
          frame "Channel2.Gain" {
            n128 = control-ref of="Deck2.Waveform"() -> (w292:refnum<vi>)
            n129 = property class="WFGraph (strict)"(reference=w292) -> (reference out=w289:refnum<vi>, "YScale.Minimum"=w291:dbl, "YScale.Maximum"=w290:dbl)  [unwired: 1 in, 1 out]
            n130 = Variant To Data(type=0.0 ("y"), Variant=w288) -> (data=w287:dbl)  [unwired: 1 in, 1 out]
            n131 = property class="WFGraph (strict)"(reference=w289, "YScale.Multiplier"=w287, "YScale.Minimum"=w291, "YScale.Maximum"=w290) -> ()  [unwired: 1 in, 2 out]
          }
        }
      }
      event Value Change {
        n132 = event-data() -> ("CtlRef"=w300:refnum<vi>, "NewVal"=w298:variant)  [unwired: 1 in, 4 out]
        n133 = property class="Ring"(reference=w300) -> (reference out=w299:refnum<vi>, "Strings []"=w296:string[])  [unwired: 1 in, 1 out]
        n134 = Variant To Data(type=u16 0, Variant=w298) -> (data=w295:u16)  [unwired: 1 in, 1 out]
        n135 = Index Array(array=w296, index=w295) -> (element=w294:string)
        n136 = call "Send UI Value Change.vi"("Data"=w294, "CtlRef"=w299) -> ()  [unwired: 10 in]
      }
      event Mouse Down? {
        # "A double-click on a numeric control (knob/slide) will reset it to its default value (usually 0 or 1). Handy for EQs!"
        n137 = event-data() -> ("CtlRef"=w305:refnum<vi>, "Button"=w307:u16, "Mods"=w306:cluster{"Double Click":bool, "Menu Key":bool})  [unwired: 1 in, 5 out]
        n138 = case shown="1" w307 {
          tunnel: w306 -> [_ w317 _]
          tunnel: w305 -> [_ w313 w333]
          tunnel: [FALSE ("Discard?") w315 TRUE ("Discard?")] -> w302
          tunnel: [w308 w314 w330] -> w304
          tunnel: w303 -> [w308 w314 _]
          frame Default {
          }
          frame 1 {
            n139 = Unbundle By Name(w317) -> ("Double Click"=w316:bool)
            n140 = property class="Ctl"(reference=w313) -> (reference out=w312:refnum<vi>, "Label.Text"=w311:string, "Value"=w310:variant)  [unwired: 1 in, 1 out]
            n141 = case shown="True" w316 {
              tunnel: [FALSE ("Discard?") TRUE ("Discard?")] -> w315
              tunnel: w312 -> [_ w319]
              tunnel: w311 -> [_ w326]
              tunnel: w310 -> [_ w324]
              frame False {
              }
              frame True {
                # "Read and written in Properties case of UI Update Loop."
                n142 = local read "Default Value Map"() -> (w323:variant)
                n143 = Get Variant Attribute(Variant=w323, name=w326, default value (empty Variant)=w324) -> (found=w325:bool, value=w322:variant)  [unwired: 1 in, 2 out]
                n144 = call "Update Control.vi"("Default Value Map"=w323, "Value In"=w322, "Control Ref"=w319) -> ("Value Out"=w321:variant, "Control Ref (Dup)"=w320:refnum<vi>)  [unwired: 5 in, 2 out]
                n145 = case shown="True" w325 {
                  tunnel: w320 -> [_ w329]
                  tunnel: w321 -> [_ w328]
                  frame False {
                  }
                  frame True {
                    n146 = property class="Ctl"(reference=w329, "Val(Sgnl)"=w328) -> ()  [unwired: 1 in, 2 out]
                  }
                }
              }
            }
          }
          frame 2 {
            # "Send a left mouse down"
            n147 = property class="Ctl"(reference=w333) -> (reference out=w332:refnum<vi>, "Value"=w331:variant)  [unwired: 1 in, 1 out]
            n148 = Bundle("CtlRef"=w332, "Value"=w331) -> (w330:cluster{"CtlRef":refnum<vi>, "Value":variant})  [unwired: 1 in]
            n149 = dll-call lib="user32.dll" fn="SendInput"("nInputs"=u32 1, "pInputs"=T13 {"type"=0, "KEYBDINPUT"={"dx"=0, "dy"=0, "mouseData"=0, "dwFlags"=2, "time"=0, "dwExtraInfo"=0}} ("input"), "cbSize"=u32 28) -> ()  [unwired: 7 in, 2 out]
          }
        }
        n150 = event-data("Discard?"=w302) -> ()  [unwired: 1 in, 1 out]
      }
      event Mouse Down {
        n151 = event-data() -> ("CtlRef"=w340:refnum<vi>, "Button"=w339:u16)  [unwired: 1 in, 6 out]
        n152 = case shown="1" w339 {
          tunnel: w340 -> [_ w343]
          frame Default {
          }
          frame 1 {
            # "When the jogwheel is clicked, send a zero move to begin scratching on a deck."
            n153 = To Variant(anything=0) -> (Variant=w341:variant)
            n154 = call "Send UI Value Change.vi"("Data"=w341, "CtlRef"=w343) -> ()  [unwired: 10 in]
          }
        }
      }
      event Value Change {
        n155 = event-data() -> ("CtlRef"=w346:refnum<vi>, "OldVal"=w350:T6, "NewVal"=w349:T6)  [unwired: 1 in, 3 out]
        n156 = call "Calculate Jogwheel Value.vi"("Playback Position"=w349) -> ("Jogwheel Label Image"=w351:i32)  [unwired: 9 in, 1 out]
        n157 = call "Calculate Jogwheel Delta.vi"("New Value"=w349, "Old Value"=w350) -> ("Delta Value"=w348:i32)  [unwired: 9 in]
        n158 = To Variant(anything=w348) -> (Variant=w347:variant)
        n159 = call "Send UI Value Change.vi"("Data"=w347, "CtlRef"=w346) -> ()  [unwired: 10 in]
        n160 = call "Parse Control Label.vi"("CtlRef"=w346) -> ("Queue Name"=w345:string)  [unwired: 9 in, 1 out]
        n161 = case shown="\"Deck2\"" w345 {
          tunnel: w351 -> [_ w352 w353]
          frame Default {
          }
          frame "Deck1" {
            "Deck1.JogwheelLabel" <- w352
          }
          frame "Deck2" {
            "Deck2.JogwheelLabel" <- w353
          }
        }
      }
      event Key Down?; event type 5.0.x8000000b; event type 1.0.x8000000b {
        # "Register Key Down events on both THIS VI (running in a sub panel), and the owning VI. Why both? Why not just the owning VI?\n\nUsing just the Key Down event from the owning VI works, EXCEPT for when the mouse is being held down at the same time. LabVIEW seems to redirect all input focus to the sub panel VI (this VI) while the mouse button is being held. As such the owning VI can no longer generate Key Down events."
        # "#BUG\nWhile holding the mouse button down on a control (moving a slider for example), F10 will not register as a key press. All other function keys seem to work.\n\nWTF.\n\nHelp mentions F3 being an issue, but that's always worked. F1 will trigger the LabVIEW help if the key press isn't discarded."
        # "#TODO\nIf file browser controls are in focus, don't execute shortcuts? Or at least allow certain key presses (arrow keys, pgup, pgdwn, home, end, etc)"
        # "Always discard the key press, and don't pass them on to controls or LabVIEW itself."
        # "Keyboard shortcuts can be setup directly on a control, but LabVIEW only supports function keys and other non-ASCII inputs. In this case we want any key to be a possible shortcut, so all key presses are captured here."
        n162 = event-data() -> ("VKey"=w356:T14, "ScanCode"=w357:i16, "Mods"=w358:cluster{"Num Pad":bool, "Menu Key":bool}, "PlatMods"=w359:T15)  [unwired: 1 in, 6 out]
        n163 = call "Parse Key Press.vi"("PlatMods"=w359, "Mods"=w358, "ScanCode"=w357, "VKey"=w356) -> ("Key Pressed"=w361:string)  [unwired: 7 in]
        n164 = Get Variant Attribute(Variant=w360, name=w361, default value (empty Variant)=T9 {"Keystroke"="", "Message Queue"="", "Event"="", "Target"="", "Data"=variant(bool FALSE)}) -> (found=w363:bool, value=w362:T9)  [unwired: 1 in, 2 out]
        n165 = case shown="True" w363 {
          tunnel: w362 -> [_ w372]
          frame False {
          }
          frame True {
            n166 = Unbundle By Name(w372) -> ("Message Queue"=w371:string, "Event"=w368:string, "Target"=w367:string, "Data"=w365:variant)
            n167 = Bundle By Name(cluster=T12 {"Event"="", "Source"="", "Target"="", "Data"=variant} ("Message"), "Event"=w368, "Target"=w367, "Data"=w365, "Source"="Shortcut") -> (w369:T12)
            n168 = call "Send.vi"("Message"=w369, "Queue Name"=w371) -> ()  [unwired: 9 in, 1 out]
          }
        }
        n169 = event-data("Discard?"=TRUE) -> ()  [unwired: 1 in, 1 out]
      }
      event Mouse Up {
        # "#NOTE\nAny changes here should be duplicated in the Mouse Up (Outside Pane) user event."
        # "Possible #BUG ?\nIf a left-mouse down is being simulated (via a right-click on a numeric), and then the right-mouse is released, a left-mouse up is simulated. LabVIEW then receives that left-mouse up and processes the command here.\n\nCould have a flag to indicate the left mouse up was simulated and ignore it?"
        n170 = event-data() -> ("Button"=w375:u16)  [unwired: 1 in, 7 out]
        n171 = case shown="1" w375 {
          tunnel: w374 -> [w376 w382 w386]
          tunnel: [w376 w382 cluster{"CtlRef":refnum<vi>, "Value":variant} {"CtlRef"=refnum, "Value"=variant}] -> w373
          frame Default {
          }
          frame 1 {
            # "#TODO\nPoll mouse buttons using Input Device Control for mouse up instead?"
            # "The Mouse Up event is sent to each deck to cancel a scratch.\n\nNote that the Mouse Up is for the entire pane (not just a jogwheel) as the mouse will more than likely NOT be over the jogwheel. This doesn't help the case where the mouse is released outside the window entirely."
            n172 = Bundle By Name(cluster=T12 {"Event"="", "Source"="", "Target"="", "Data"=variant} ("Message"), "Event"="Mouse Up" ("Type")) -> (w377:T12)
            n173 = call "Send.vi"("Message"=w377, "Queue Name"="Deck1") -> ()  [unwired: 9 in, 1 out]
            n174 = call "Send.vi"("Message"=w377, "Queue Name"="Deck2") -> ()  [unwired: 9 in, 1 out]
          }
          frame 2 {
            n175 = Unbundle(w386) -> ("CtlRef"=w384:refnum<vi>, "Value"=w383:variant)
            n176 = Not A Number/Path/Refnum?(number/path/refnum=w384) -> (NaN/Path/Refnum?=w385:bool)
            n177 = case shown="False" w385 {
              tunnel: w384 -> [w389 _]
              tunnel: w383 -> [w388 _]
              frame False {
                # "Send a left mouse up"
                # "Reset the value"
                n178 = property class="Ctl"(reference=w389, "Val(Sgnl)"=w388) -> ()  [unwired: 1 in, 2 out]
                n179 = dll-call lib="user32.dll" fn="SendInput"("nInputs"=u32 1, "pInputs"=T13 {"type"=0, "KEYBDINPUT"={"dx"=0, "dy"=0, "mouseData"=0, "dwFlags"=4, "time"=0, "dwExtraInfo"=0}} ("input"), "cbSize"=u32 28) -> ()  [unwired: 7 in, 2 out]
              }
              frame True {
              }
            }
          }
        }
      }
      event Mouse Enter {
        w393 = FALSE ("Visible")
        n180 = event-data() -> ()  [unwired: 1 in, 4 out]
        n181 = property on="Deck1.DragDropPath" class="Path"("Visible"=w393) -> ()  [unwired: 2 in, 2 out]
        n182 = property on="Deck2.DragDropPath" class="Path"("Visible"=w393) -> ()  [unwired: 2 in, 2 out]
      }
      event Mouse Leave {
        w395 = TRUE ("Visible")
        n183 = event-data() -> ()  [unwired: 1 in, 4 out]
        n184 = property on="Deck1.DragDropPath" class="Path"("Visible"=w395) -> ()  [unwired: 2 in, 2 out]
        n185 = property on="Deck2.DragDropPath" class="Path"("Visible"=w395) -> ()  [unwired: 2 in, 2 out]
      }
    }
  }
  n186 = Unregister For Events(event registration refnum=w30) -> ()  [unwired: 1 in, 1 out]
  n187 = Release Queue(queue=w19, force destroy? (F)=TRUE, error in (no error)=w26) -> ()  [unwired: 3 out]
